vi "Drag & Drop End Multi.vi"(8 "errorin":errorcluster, 11 "References In":T1(array[cluster])) -> (0 "error out":errorcluster)   [LabVIEW 2015]
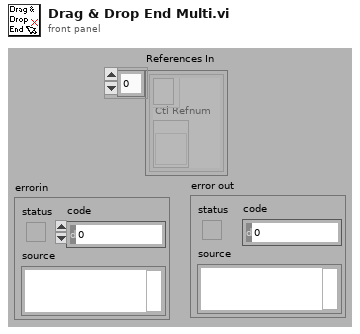
[diagram p1: front panel]
types:
  T1 = cluster{"Event Registration Refnum":refnum<event-registration>, "Ctl Refnum":refnum<vi>}[]
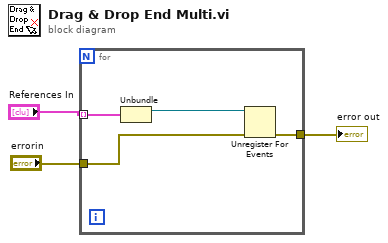
[diagram p0: block diagram]
diagram:
  n1 = for {
    tunnel: [w6] -> w2
    tunnel: "errorin" -> [w5]
    tunnel: "References In" -> [w4] mode=indexing
    n2 = Unbundle(w4) -> ("Event Registration Refnum"=w7:refnum<event-registration>)  [unwired: 1 out]
    n3 = Unregister For Events(event registration refnum=w7, error in=w5) -> (error out=w6:errorcluster)
  }
  "error out" <- w2
